vi "Handle Variable Header.vi"(8 "error in (no error)":errorcluster, 10 "Incoming Packets":u8[](array[numeric]) format="%08b", 11 "PUBLISH in":refnum<class "PUBLISH.lvclass">) -> (0 "error out":errorcluster, 1 "Variable Header Complete?":bool=TRUE, 2 "Remaining Packets":u8[](array[numeric]) format="%08b", 3 "PUBLISH out":refnum<class "PUBLISH.lvclass">)   [LabVIEW 2013, in "PUBLISH.lvclass"]
uses:
  PUBLISH.lvclass
  ControlPacket/ControlPacket.lvclass/ControlPacket.ctl
  ControlPacket/ControlPacket.lvclass
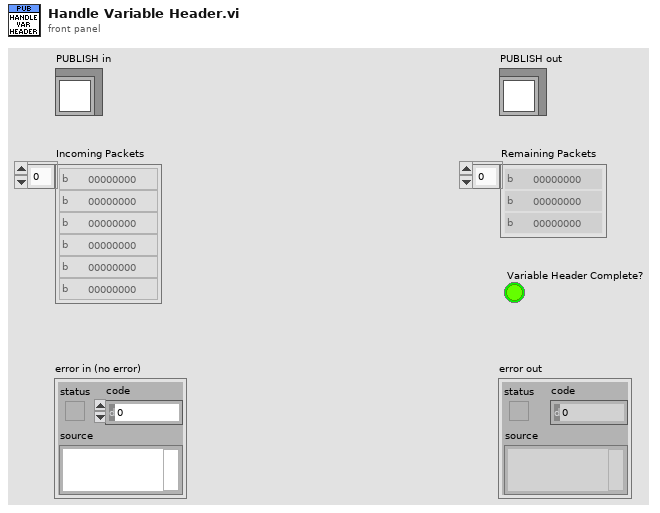
[diagram p1: front panel]
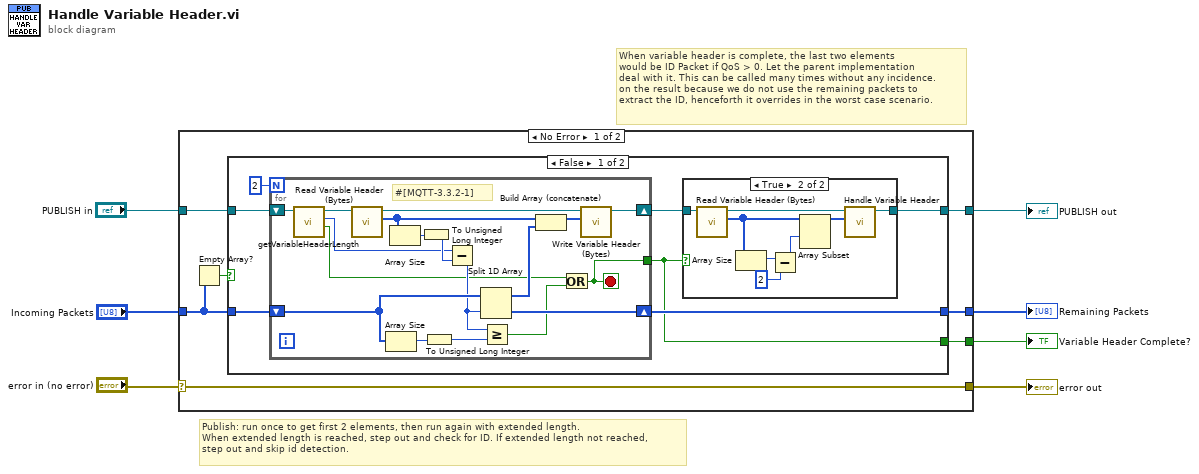
[diagram p0: block diagram]
diagram:
  # "When variable header is complete, the last two elements\nwould be ID Packet if QoS > 0. Let the parent implementation\ndeal with it. This can be called many times without any incidence.\non the result because we do not use the remaining packets to\nextract the ID, henceforth it overrides in the worst case scenario."
  # "Publish: run once to get first 2 elements, then run again with extended length.\nWhen extended length is reached, step out and check for ID. If extended length not reached,\nstep out and skip id detection."
  n1 = case shown="No Error" "error in (no error)" {
    selector: "error in (no error)" -> [w10 w51]
    tunnel: "PUBLISH in" -> [w14 w53]
    tunnel: "Incoming Packets" -> [w9 w52]
    tunnel: [w13 _] -> w3
    tunnel: [w12 w52] -> w2
    tunnel: [w11 w53] -> w1
    tunnel: [w10 w51] -> w4
    frame No Error {
      n2 = Empty Array?(array=w9) -> (empty?=w8:bool)
      n3 = case shown="False" w8 {
        tunnel: w14 -> [w21 w50]
        tunnel: [w15 _] -> w13
        tunnel: [w20 w49] -> w12
        tunnel: [w17 w50] -> w11
        tunnel: w9 -> [w19 w49]
        frame False {
          n4 = for {
            N: 2 -> [_]
            tunnel: [w31] -> w15
            shift-right: [w37] -> w20
            shift-left: w19 -> [w41]
            shift-right: [w36] -> w16
            shift-left: w21 -> [w46]
            stop <- w31 stop-if-true
            # "#[MQTT-3.3.2-1]"
            n5 = call-dynamic "getVariableHeaderLength.vi"("PUBLISH in"=w46) -> ("size definitive"=w32:bool, "VariableHeader size"=w35:u32, "PUBLISH out"=w48:refnum<class "PUBLISH.lvclass">)  [unwired: 8 in]
            n6 = call "Read Variable Header (Bytes).vi"("ControlPacket in"=w48) -> ("Variable Header (Bytes)"=w34:u8[], "ControlPacket out"=w47:refnum<class "PUBLISH.lvclass">)  [unwired: 9 in]
            n7 = Array Size(array=w41) -> (size(s)=w40:i32)
            n8 = Array Size(array=w34) -> (size(s)=w45:i32)
            n9 = To Unsigned Long Integer(number=w45) -> (unsigned 32bit integer=w42:u32)
            n10 = To Unsigned Long Integer(number=w40) -> (unsigned 32bit integer=w39:u32)
            n11 = Subtract(x=w35, y=w42) -> (x-y=w38:u32)
            n12 = Split 1D Array(array=w41, index=w38) -> (first subarray=w44:u8[], second subarray=w37:u8[])
            n13 = Greater Or Equal?(x=w38, y=w39) -> (x >= y?=w33:bool)
            n14 = Build Array (concatenate)(w34, w44) -> (w43:u8[])
            n15 = Or(x=w32, y=w33) -> (x .or. y?=w31:bool)
            n16 = call "Write Variable Header (Bytes).vi"("Variable Header (Bytes)"=w43, "ControlPacket in"=w47) -> ("ControlPacket out"=w36:refnum<class "PUBLISH.lvclass">)  [unwired: 9 in]
          }
          n17 = case shown="True" w15 {
            tunnel: [w22 w30] -> w17
            tunnel: w16 -> [w22 w29]
            frame False {
            }
            frame True {
              n18 = call "Read Variable Header (Bytes).vi"("ControlPacket in"=w29) -> ("Variable Header (Bytes)"=w27:u8[], "ControlPacket out"=w28:refnum<class "PUBLISH.lvclass">)  [unwired: 9 in]
              n19 = Array Size(array=w27) -> (size(s)=w25:i32)
              n20 = Subtract(x=w25, y=2) -> (x-y=w23:i32)
              n21 = Array Subset(array=w27, index=w23) -> (w26:u8[])  [unwired: 1 in]
              n22 = call-parent "Handle Variable Header.vi"("Incoming Packets"=w26, "ControlPacket in"=w28) -> ("ControlPacket out"=w30:refnum<class "PUBLISH.lvclass">)  [unwired: 6 in, 3 out]
            }
          }
        }
        frame True {
        }
      }
    }
    frame Error {
    }
  }
  "error out" <- w4
  "PUBLISH out" <- w1
  "Remaining Packets" <- w2
  "Variable Header Complete?" <- w3
